vi "LoadWeighting.vi"() -> ()   [LabVIEW 2012]
uses:
  <vilib>/Utility/file.llb/Read From Spreadsheet File (string).vi
  <vilib>/addons/database/Connection.llb/DB Tools Open Connec (Path).vi
  <vilib>/addons/database/Connection.llb/Conn Execute.vi
  <vilib>/addons/database/Recordset.llb/Rec Fetch Integer Data (R).vi
  <vilib>/addons/database/Recordset.llb/Rec Destroy - Connection.vi
  <vilib>/addons/database/NI_Database_API.lvlib
panel:
  in  "connection information":path=path "C:/m100/data/m100.dsn"
  out "error out":errorcluster
  out "output cluster":T1
  in  "Cluster":T1
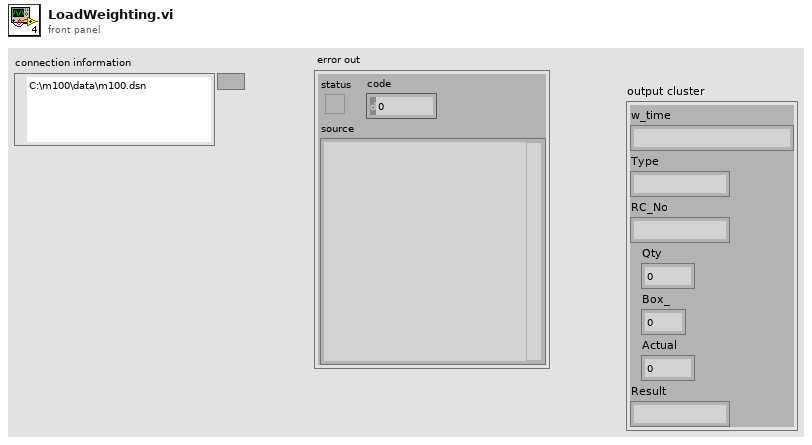
[diagram p1: front panel]
types:
  T1 = cluster{"w_time":string, "Type":string, "RC_No":string, "Qty":dbl, "Box_":dbl, "Actual":dbl, "Result":string}
  T2 = typedef "NI_Database_API.lvlib/Conn ObjectReference.ctl" = refnum<k1>
  T3 = typedef "NI_Database_API.lvlib/Rec ObjectReference.ctl" = refnum<k1>
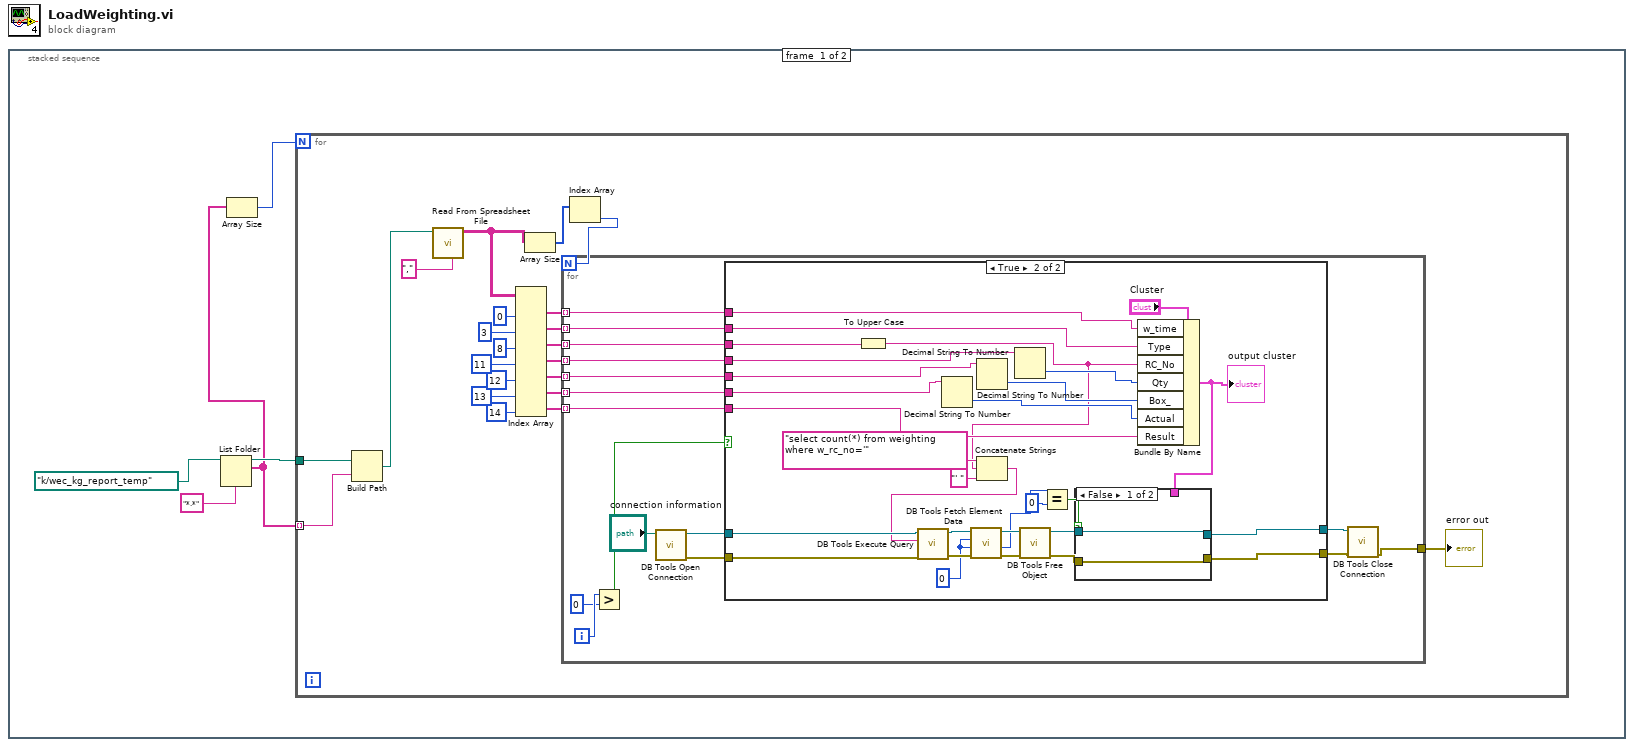
[diagram p0: block diagram]
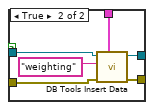
[diagram p3: hidden frame]
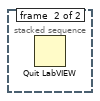
[diagram p4: hidden frame]
diagram:
  n1 = stacked-sequence {
    frame #0 {
      n2 = List Folder(path=path "k:/wec_kg_report_temp", pattern="*.*") -> (path out=w3:path, filenames=w1:string[])  [unwired: 2 in, 2 out]
      n3 = Array Size(array=w1) -> (size(s)=w2:i32)
      n4 = for {
        N: w2 -> [_]
        tunnel: w3 -> [w8]
        tunnel: w1 -> [w6] mode=indexing
        n5 = Build Path(base path=w8, name or relative path=w6) -> (appended path=w7:path)
        n6 = call-poly <vilib>:"Read From Spreadsheet File.vi"("delimiter (\\t)"="," ("delimiter (\\t)"), "file path (dialog if empty)"=w7) -> ("all rows"=w25:string[][])  [unwired: 5 in, 4 out]
        n7 = Index Array(array=w25, index (col) #1=0 ("disabled index (col)"), index (col) #2=3 ("index (col)"), index (col) #3=8 ("index (col)"), index (col) #4=11 ("index (col)"), index (col) #5=12 ("index (col)"), index (col) #6=13 ("index (col)"), index (col) #7=14 ("index (col)")) -> (element #1=w17:string[], element #2=w15:string[], element #3=w14:string[], element #4=w13:string[], element #5=w12:string[], element #6=w11:string[], element #7=w10:string[])  [unwired: 7 in]
        n8 = Array Size(array=w25) -> (size(s)=w26:i32[])
        n9 = Index Array(array=w26) -> (element=w16:i32)  [unwired: 1 in]
        n10 = for {
          N: w16 -> [_]
          tunnel: w17 -> [w40] mode=indexing
          tunnel: w15 -> [w39] mode=indexing
          tunnel: w14 -> [w38] mode=indexing
          tunnel: w13 -> [w37] mode=indexing
          tunnel: w12 -> [w36] mode=indexing
          tunnel: w11 -> [w35] mode=indexing
          tunnel: w10 -> [w34] mode=indexing
          tunnel: [w29] -> w9
          i -> [w42]
          n11 = Greater?(x=w42, y=0) -> (0:w43:bool)
          n12 = call-poly <vilib>:"DB Tools Open Connection.vi"("connection information"="connection information") -> ("error out"=w32:errorcluster, "connection reference"=w33:T2)  [unwired: 7 in]
          n13 = case shown="True" w43 {
            tunnel: w40 -> [_ w74]
            tunnel: w39 -> [_ w73]
            tunnel: w38 -> [_ w47]
            tunnel: w37 -> [_ w72]
            tunnel: w36 -> [_ w70]
            tunnel: w35 -> [_ w68]
            tunnel: w34 -> [_ w66]
            tunnel: w33 -> [w45 w62]
            tunnel: w32 -> [w44 w61]
            tunnel: [w45 w65] -> w31
            tunnel: [w44 w64] -> w30
            frame False {
            }
            frame True {
              w48 = 0
              n14 = To Upper Case(1:w47) -> (0:w46:string)
              n15 = Decimal String To Number(string=w68) -> (number=w67:i32)  [unwired: 2 in, 1 out]
              n16 = Decimal String To Number(string=w70) -> (number=w69:i32)  [unwired: 2 in, 1 out]
              n17 = Concatenate Strings("select count(*) from weighting where w_rc_no='" ("string"), w46, "' " ("string")) -> (w52:string)
              n18 = call-poly <vilib>:"DB Tools Execute Query.vi"("error in (no error)"=w61, "SQL query"=w52, "connection reference"=w62) -> ("error out"=w58:errorcluster, "recordset reference"=w59:T3)  [unwired: 5 in]
              n19 = call-poly <vilib>:"DB Tools Fetch Element Data.vi"("error in (no error)"=w58, "type"=w48, "column index"=w48, "recordset reference"=w59) -> ("error out"=w60:errorcluster, "data"=w51:i32, "recordset reference out"=w57:T3)  [unwired: 3 in]
              n20 = Decimal String To Number(string=w72) -> (number=w71:i32)  [unwired: 2 in, 1 out]
              n21 = call-poly <vilib>:"DB Tools Free Object.vi"("error in (no error)"=w60, "recordset reference"=w57) -> ("error out"=w55:errorcluster, "connection reference"=w56:T2)  [unwired: 8 in]
              n22 = Equal?(x=w51, y=0) -> (x = y?=w49:bool)
              n23 = Bundle By Name(cluster="Cluster", "w_time"=w74, "Type"=w73, "RC_No"=w46, "Qty"=w71, "Box_"=w69, "Actual"=w67, "Result"=w66) -> (w63:T1)
              "output cluster" <- w63
              n24 = case shown="False" w49 {
                tunnel: [w77 w83] -> w65
                tunnel: [w76 w82] -> w64
                tunnel: w63 -> [_ w80]
                tunnel: w56 -> [w77 w79]
                tunnel: w55 -> [w76 w78]
                frame False {
                }
                frame True {
                  n25 = call <vilib>:"DB Tools Insert Data.vi"("data"=w80, "error in (no error)"=w78, "table"="weighting", "connection reference"=w79) -> ("error out"=w82:errorcluster, "connection reference out"=w83:T2)  [unwired: 6 in]
                }
              }
            }
          }
          n26 = call <vilib>:"DB Tools Close Connection.vi"("error in (no error)"=w30, "connection reference"=w31) -> ("error out"=w29:errorcluster)  [unwired: 5 in]
        }
        "error out" <- w9
      }
    }
    frame #1 {
      n27 = Quit LabVIEW() -> ()  [unwired: 1 in]
    }
  }
